vi "connect_visa_write_wires.vi"(0 "Terms[]":refnum<vi>[](array[refnum]), 1 "Last StrCnst Refnum":refnum<vi>, 5 "Last Function":refnum<vi>, 7 "VISA In Term":refnum<vi>, 9 "Error In Term":refnum<vi>, 11 "error in":errorcluster) -> (8 "Visa Out Term":refnum<vi>, 10 "Error Out Term":refnum<vi>, 15 "error out":errorcluster)   [LabVIEW 2018]
uses:
  Iternl/ConttWire/TypeDefines/connect_with_last_node_types.ctl
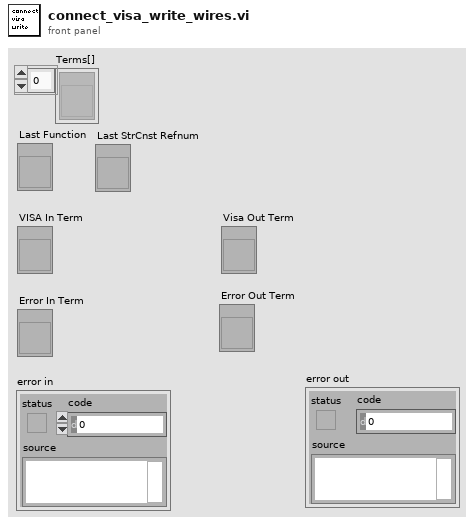
[diagram p1: front panel]
types:
  T1 = typedef "connect_with_last_node_types.ctl" = u16
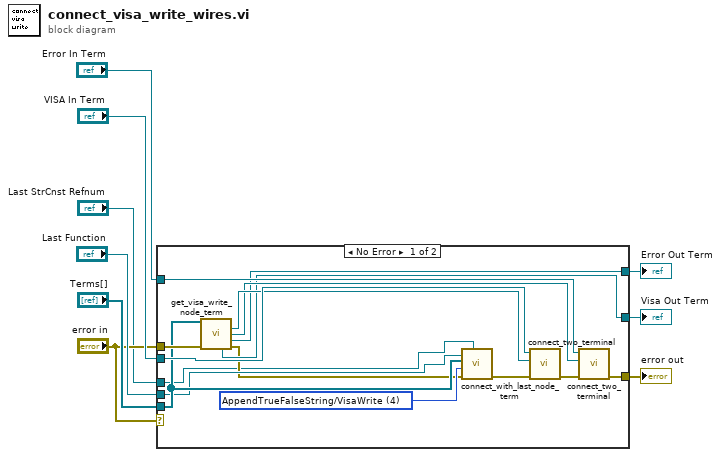
[diagram p0: block diagram]
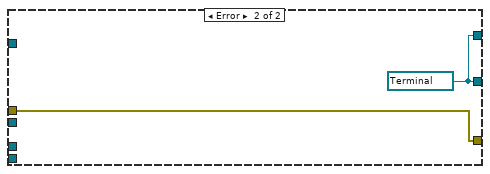
[diagram p2: hidden frame]
diagram:
  n1 = case shown="No Error" "error in" {
    tunnel: "error in" -> [w24 w26]
    tunnel: "VISA In Term" -> [w23 _]
    tunnel: "Error In Term" -> [w20 _]
    tunnel: [w19 w25] -> w7
    tunnel: [w18 w25] -> w6
    tunnel: "Terms[]" -> [w16 _]
    tunnel: "Last Function" -> [w14 _]
    tunnel: [w11 w26] -> w2
    tunnel: "Last StrCnst Refnum" -> [w10 _]
    frame No Error {
      w15 = T1 4 items=["AppendTrueFalseString/VisaWrite"=4, "PickLine"=3, "FormatIntoString"=1] ("Terminal Index")
      n2 = call "get_visa_write_node_term.vi"("Terms[] In"=w16, "error in (no error)"=w24) -> ("VISA In  Term"=w22:refnum<vi>, "Error In Term"=w21:refnum<vi>, "Error Out Term"=w18:refnum<vi>, "Visa Out Term"=w19:refnum<vi>, "error out"=w12:errorcluster)  [unwired: 9 out]
      n3 = call "connect_with_last_node_term.vi"("Last StrCnst Refnum"=w10, "error in (no error)"=w12, "Terminal Index"=w15, "Terminals[]"=w16, "Last Function Ref In"=w14) -> ("error out"=w13:errorcluster)  [unwired: 6 out]
      n4 = call "connect_two_terminal.vi"("error in"=w13, "Terminal 2"=w22, "Terminal 1"=w23) -> ("error out"=w17:errorcluster)  [unwired: 1 in, 7 out]
      n5 = call "connect_two_terminal.vi"("error in"=w17, "Terminal 2"=w21, "Terminal 1"=w20) -> ("error out"=w11:errorcluster)  [unwired: 1 in, 7 out]
    }
    frame Error {
      w25 = refnum<vi> refnum ("Error Out Term")
    }
  }
  "Visa Out Term" <- w7
  "Error Out Term" <- w6
  "error out" <- w2
